vi "temperatury.vi"() -> ()   [LabVIEW 2018]
panel:
  out "String":string
  in  "Target scale":enum16{"Celsius", "Kelvin", "Fahrenheit"}(ring)
  in  "Present scale":enum16{"Celsius", "Kelvin", "Fahrenheit"}(ring)
  in  "Temperature":dbl
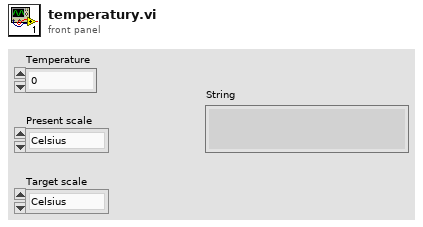
[diagram p1: front panel]
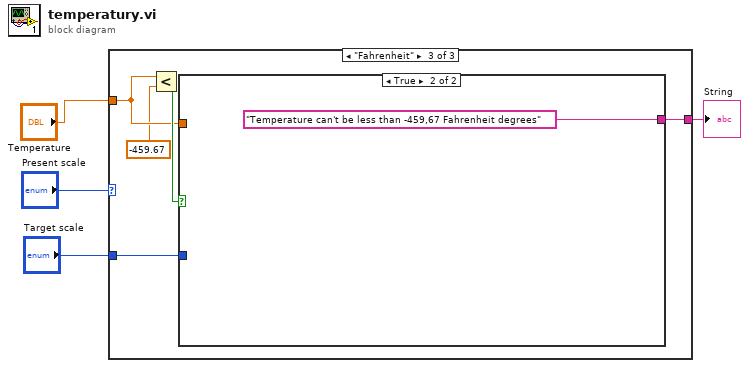
[diagram p0: block diagram]
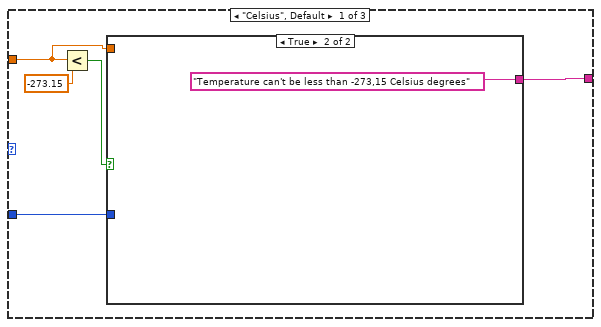
[diagram p2: hidden frame]
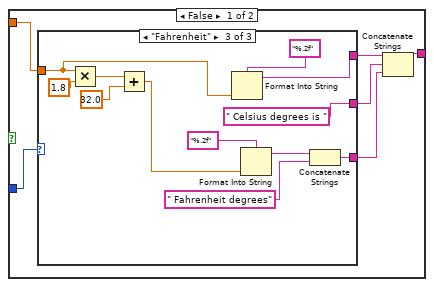
[diagram p3: hidden frame]
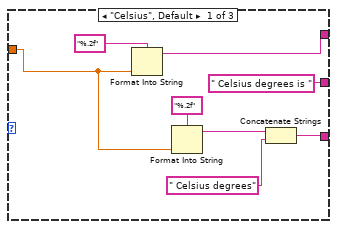
[diagram p4: hidden frame]
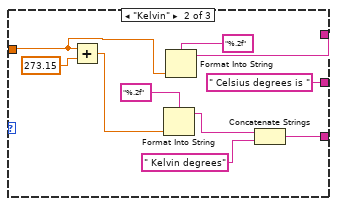
[diagram p5: hidden frame]
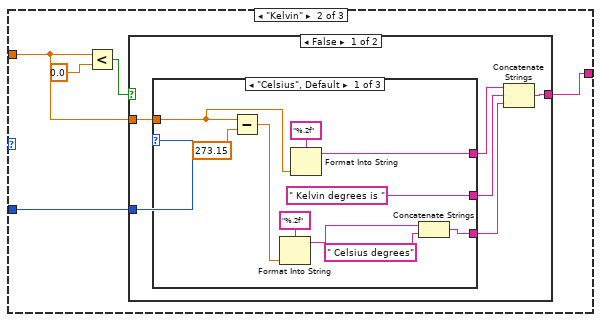
[diagram p6: hidden frame]
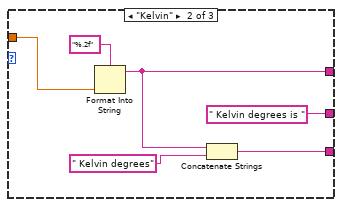
[diagram p7: hidden frame]
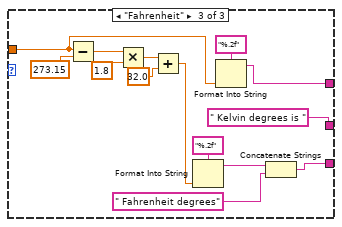
[diagram p8: hidden frame]
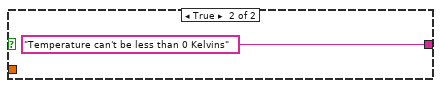
[diagram p9: hidden frame]
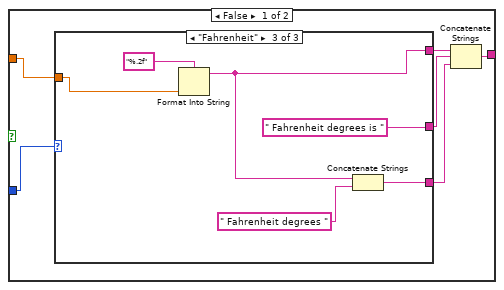
[diagram p10: hidden frame]
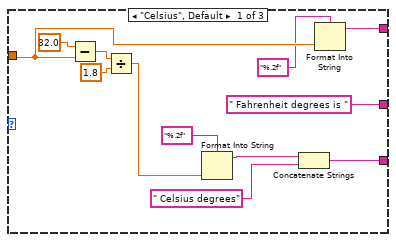
[diagram p11: hidden frame]
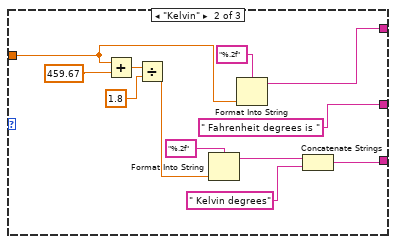
[diagram p12: hidden frame]
diagram:
  n1 = case shown="\"Fahrenheit\"" "Present scale" {
    tunnel: "Temperature" -> [w5 w47 w90]
    tunnel: [w7 w49 w93] -> w2
    tunnel: "Target scale" -> [w6 w48 w92]
    frame "Celsius", Default {
      n2 = Less?(x=w5, y=-273.15) -> (x < y?=w8:bool)
      n3 = case shown="True" w8 {
        tunnel: [w13 "Temperature can't be less than -273,15 Celsius degrees"] -> w7
        tunnel: w6 -> [w15 _]
        tunnel: w5 -> [w14 _]
        frame False {
          n4 = case shown="\"Fahrenheit\"" w15 {
            tunnel: w14 -> [w21 w30 w40]
            tunnel: [w23 w32 w42] -> w12
            tunnel: [" Celsius degrees is " " Celsius degrees is " " Celsius degrees is "] -> w11
            tunnel: [w19 w26 w38] -> w10
            frame "Celsius", Default {
              n5 = Format Into String(format string="%.2f", w21) -> (resulting string=w23:string)  [unwired: 2 in, 1 out]
              n6 = Format Into String(format string="%.2f", w21) -> (resulting string=w20:string)  [unwired: 2 in, 1 out]
              n7 = Concatenate Strings(w20, " Celsius degrees") -> (w19:string)
            }
            frame "Kelvin" {
              n8 = Add(x=w30, y=273.15 ("x")) -> (x+y=w29:dbl)
              n9 = Format Into String(format string="%.2f", w29) -> (resulting string=w27:string)  [unwired: 2 in, 1 out]
              n10 = Format Into String(format string="%.2f", w30) -> (resulting string=w32:string)  [unwired: 2 in, 1 out]
              n11 = Concatenate Strings(w27, " Kelvin degrees") -> (w26:string)
            }
            frame "Fahrenheit" {
              n12 = Multiply(x=w40, y=1.8) -> (x*y=w44:dbl)
              n13 = Add(x=w44, y=32.0) -> (x+y=w39:dbl)
              n14 = Format Into String(format string="%.2f", w40) -> (resulting string=w42:string)  [unwired: 2 in, 1 out]
              n15 = Format Into String(format string="%.2f", w39) -> (resulting string=w37:string)  [unwired: 2 in, 1 out]
              n16 = Concatenate Strings(w37, " Fahrenheit degrees") -> (w38:string)
            }
          }
          n17 = Concatenate Strings(w12, w11, w10) -> (w13:string)
        }
        frame True {
        }
      }
    }
    frame "Kelvin" {
      n18 = Less?(x=w47, y=0.0) -> (x < y?=w50:bool)
      n19 = case shown="False" w50 {
        tunnel: [w52 "Temperature can't be less than 0 Kelvins"] -> w49
        tunnel: w48 -> [w57 _]
        tunnel: w47 -> [w56 _]
        frame False {
          n20 = case shown="\"Celsius\", Default" w57 {
            tunnel: w56 -> [w65 w73 w82]
            tunnel: [w64 w72 w81] -> w55
            tunnel: [" Kelvin degrees is " " Kelvin degrees is " " Kelvin degrees is "] -> w54
            tunnel: [w61 w70 w78] -> w53
            frame "Celsius", Default {
              n21 = Subtract(x=w65, y=273.15) -> (x-y=w66:dbl)
              n22 = Format Into String(format string="%.2f", w66) -> (resulting string=w62:string)  [unwired: 2 in, 1 out]
              n23 = Format Into String(format string="%.2f", w65) -> (resulting string=w64:string)  [unwired: 2 in, 1 out]
              n24 = Concatenate Strings(w62, " Celsius degrees") -> (w61:string)
            }
            frame "Kelvin" {
              n25 = Format Into String(format string="%.2f" ("resulting string"), w73) -> (resulting string=w72:string)  [unwired: 2 in, 1 out]
              n26 = Concatenate Strings(w72, " Kelvin degrees") -> (w70:string)
            }
            frame "Fahrenheit" {
              n27 = Subtract(x=w82, y=273.15) -> (x-y=w86:dbl)
              n28 = Multiply(x=w86, y=1.8) -> (x*y=w84:dbl)
              n29 = Add(x=w84, y=32.0) -> (x+y=w79:dbl)
              n30 = Format Into String(format string="%.2f", w79) -> (resulting string=w77:string)  [unwired: 2 in, 1 out]
              n31 = Format Into String(format string="%.2f", w82) -> (resulting string=w81:string)  [unwired: 2 in, 1 out]
              n32 = Concatenate Strings(w77, " Fahrenheit degrees") -> (w78:string)
            }
          }
          n33 = Concatenate Strings(w55, w54, w53) -> (w52:string)
        }
        frame True {
        }
      }
    }
    frame "Fahrenheit" {
      n34 = Less?(x=w90, y=-459.67) -> (x < y?=w91:bool)
      n35 = case shown="True" w91 {
        tunnel: [w97 "Temperature can't be less than -459,67 Fahrenheit degrees"] -> w93
        tunnel: w90 -> [w98 _]
        tunnel: w92 -> [w99 _]
        frame False {
          n36 = case shown="\"Fahrenheit\"" w99 {
            tunnel: w98 -> [w108 w121 w129]
            tunnel: [" Fahrenheit degrees is " " Fahrenheit degrees is " " Fahrenheit degrees is "] -> w96
            tunnel: [w105 w117 w127] -> w95
            tunnel: [w104 w122 w126] -> w94
            frame "Celsius", Default {
              n37 = Subtract(x=32.0 ("x-y"), y=w108) -> (x-y=w110:dbl)
              n38 = Divide(x=w110, y=1.8 ("x/y")) -> (x/y=w106:dbl)
              n39 = Format Into String(format string="%.2f", w106) -> (resulting string=w103:string)  [unwired: 2 in, 1 out]
              n40 = Concatenate Strings(w103, " Celsius degrees") -> (w105:string)
              n41 = Format Into String(format string="%.2f", w108) -> (resulting string=w104:string)  [unwired: 2 in, 1 out]
            }
            frame "Kelvin" {
              n42 = Add(x=w121, y=459.67) -> (x+y=w120:dbl)
              n43 = Divide(x=w120, y=1.8 ("x/y")) -> (x/y=w116:dbl)
              n44 = Format Into String(format string="%.2f", w116) -> (resulting string=w115:string)  [unwired: 2 in, 1 out]
              n45 = Format Into String(format string="%.2f", w121) -> (resulting string=w122:string)  [unwired: 2 in, 1 out]
              n46 = Concatenate Strings(w115, " Kelvin degrees") -> (w117:string)
            }
            frame "Fahrenheit" {
              n47 = Format Into String(format string="%.2f", w129) -> (resulting string=w126:string)  [unwired: 2 in, 1 out]
              n48 = Concatenate Strings(w126, " Fahrenheit degrees ") -> (w127:string)
            }
          }
          n49 = Concatenate Strings(w94, w96, w95) -> (w97:string)
        }
        frame True {
        }
      }
    }
  }
  "String" <- w2
